vi "Register gRPC Methods.vi"(8 "error in (no error)":errorcluster, 11 "Template Server in":refnum<class "Query Server.lvclass">) -> (0 "error out":errorcluster, 3 "Template Server out":refnum<class "Query Server.lvclass">)   [LabVIEW 2019, in "Query Server.lvlib" / "Query Server.lvclass"]
uses:
  Query Server.lvclass
  typeDefs/Server Internal UEs.ctl
  typeDefs/Server Internal Message.ctl
  typeDefs/Server gRPC UEs.ctl
  gRPC lvSupport/Server API/typeDefs/gRPCId Cluster.ctl
  gRPC lvSupport/Server API/typeDefs/grpcId.ctl
  Query Server.lvclass/Query Server.ctl
  gRPC lvSupport/gprc-lvsupport.lvlib
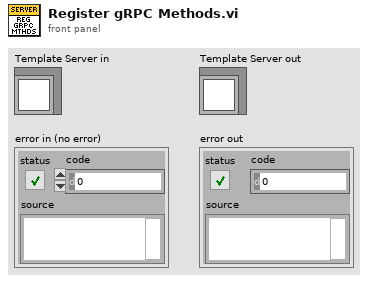
[diagram p1: front panel]
types:
  T1 = typedef "Query Server.lvlib/Query Server.lvclass/Server gRPC UEs.ctl" = cluster{"Invoke gRPC UE":refnum<user-event>, "Query gRPC UE":refnum<user-event>, "Register gRPC UE":refnum<user-event>}
  T2 = typedef "Query Server.lvlib/Query Server.lvclass/Server Internal UEs.ctl" = cluster{"Invoke Internal UE":refnum<user-event>, "Query Internal UE":refnum<user-event>, "Register Internal UE":refnum<user-event>}
  T3 = typedef "Query Server.lvlib/gprc-lvsupport.lvlib/grpcId.ctl" = u64
  T4 = typedef "Query Server.lvlib/Query Server.lvclass/Server Internal Message UE.ctl" = refnum<user-event>
  T5 = typedef "Query Server.lvlib/gprc-lvsupport.lvlib/gRPCId Cluster UE.ctl" = refnum<user-event>
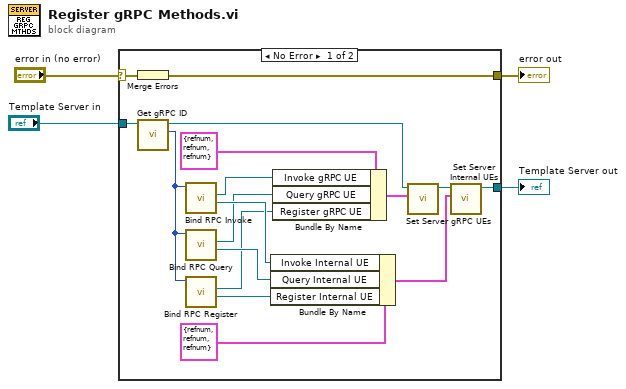
[diagram p0: block diagram]
diagram:
  n1 = case shown="No Error" "error in (no error)" {
    selector: "error in (no error)" -> [w12 w22]
    tunnel: "Template Server in" -> [w20 w23]
    tunnel: [w19 w22] -> w3
    tunnel: [w18 w23] -> w2
    frame No Error {
      n2 = Merge Errors(w12) -> (w19:errorcluster)
      n3 = call "Get gRPC ID.vi"("OOP Server in"=w20) -> ("gRPC ID"=w11:T3, "OOP Server out"=w21:refnum<class "Query Server.lvclass">)  [unwired: 9 in]
      n4 = call "Bind RPC Invoke.vi"("gRPCid server in"=w11) -> ("Invoke Internal UE"=w10:T4, "Invoke gRPC UE"=w9:T5)  [unwired: 7 in, 2 out]
      n5 = call "Bind RPC Query.vi"("gRPCid server in"=w11) -> ("Query Internal UE"=w8:T4, "Query gRPC UE"=w7:T5)  [unwired: 7 in, 2 out]
      n6 = call "Bind RPC Register.vi"("gRPCid server in"=w11) -> ("Register Internal UE"=w6:T4, "Register gRPC UE"=w5:T5)  [unwired: 7 in, 2 out]
      n7 = Bundle By Name ("Bundle Internal UEs")(cluster=T2 {"Invoke Internal UE"=refnum, "Query Internal UE"=refnum, "Register Internal UE"=refnum} ("Server Internal UEs"), "Invoke Internal UE"=w10, "Query Internal UE"=w8, "Register Internal UE"=w6) -> (w17:T2)
      n8 = Bundle By Name ("Bundle gRPC UEs")(cluster=T1 {"Invoke gRPC UE"=refnum, "Query gRPC UE"=refnum, "Register gRPC UE"=refnum} ("gRPC Server Method Events"), "Invoke gRPC UE"=w9, "Query gRPC UE"=w7, "Register gRPC UE"=w5) -> (w14:T1)
      n9 = call "Set Server gRPC UEs.vi"("Server gRPC UEs"=w14, "OOP Server in"=w21) -> ("OOP Server out"=w15:refnum<class "Query Server.lvclass">)  [unwired: 9 in]
      n10 = call "Set Server Internal UEs.vi"("Server Internal UEs"=w17, "OOP Server in"=w15) -> ("OOP Server out"=w18:refnum<class "Query Server.lvclass">)  [unwired: 9 in]
    }
    frame Error {
    }
  }
  "error out" <- w3
  "Template Server out" <- w2
